vi "Basic Example.vi"(11 "System Definition Configuration":T34={"System Definition Path"=path "C:/Users/Public/Documents/National Instruments/NI VeriStand 2024/Projects/SimpleSystemDef Example/SimpleSystemDef.nivssdf", "Targets"=[{"Target Settings"={"Name"="Controller", "Target Type"="Windows", "IPAddress"="localhost", "PrimaryControlLoopProcessor"=-2, "DataProcessingLoopProcessor"=-2, "DataProcessingLoopDecimation"=1, "DAQDigitalLinesDecimation"=1, "MaximumStreamedChannels"=512, "ExecutionMode"=0, "FilterDAQErrors"=FALSE, "FilterWatchdogErrors"=FALSE, "FPGAScanInterfaceMode"=0, "TargetRate"=100.0}, "Chassises"=[{"Chassis Settings"={"Name"="Controller", "Master Chassis"={"Type"=enum."None", "DAQ Name"="", "clkSrc"=0, "activeEdge"=10280, "exportClk"=0, "exportClkToLine"=0, "triggerLine"=10171, "triggerSlope"=0, "startTrigger"=0, "startTriggerLine"=0}}, "DAQ Boards"=[{"Name"="DAQ1", "Description"="", "InputConfiguration"=10106, "TurnOffHWTimedSinglePointAI"=FALSE, "TurnOffHWTimedSinglePointAO"=FALSE, "DAQConversionRateOption"=0, "PortWidth"=8, "Analog Inputs"=[{"Name"="DAN0", "Units"="V", "InitialValue"=0.0, "HighLevel"=10.0, "LowLevel"=-10.0, "Channel"=0, "ChannelType"=0, "Alias Name"=""}, {"Name"="DAN1", "Units"="V", "InitialValue"=0.0, "HighLevel"=10.0, "LowLevel"=-10.0, "Channel"=1, "ChannelType"=0, "Alias Name"=""}], "Analog Outputs"=[{"Name"="DON0", "Units"="V", "InitialValue"=0.0, "HighLevel"=10.0, "LowLevel"=-10.0, "Channel"=0, "ChannelType"=0, "Alias Name"=""}, {"Name"="DON1", "Units"="V", "InitialValue"=0.0, "HighLevel"=10.0, "LowLevel"=-10.0, "Channel"=1, "ChannelType"=0, "Alias Name"=""}], "DIO Port Settings"=[{"portNumber"=0, "Inverted"=FALSE, "Digital Inputs"=[{"Name"="DIN0", "InitialValue"=FALSE, "DigitalLine"=0, "Alias Name"=""}, {"Name"="DIN1", "InitialValue"=FALSE, "DigitalLine"=2, "Alias Name"=""}], "Digital Outputs"=[{"Name"="DUN0", "InitialValue"=FALSE, "DigitalLine"=1, "Alias Name"=""}, {"Name"="DUN1", "InitialValue"=FALSE, "DigitalLine"=3, "Alias Name"=""}]}], "Counter Settings"={"Frequency Measurements"=[], "Period Measurements"=[], "Count Measurements"=[], "Position Measurements"=[]}}], "FPGA Boards"=[], "CAN Boards"=[]}], "Custom Devices"=[], "Models"=[], "User Channels"=[], "Calculated Channels"={"Formula Settings"=[], "Average Settings"=[], "Acceleration Settings"=[], "Maximum Settings"=[], "Minimum Settings"=[], "Peak and Valley Settings"=[], "Conditional Settings"=[]}, "Alarms"=[]}], "Aliases"=[], "System Mappings"={"Mapping Pairs"=[]}} {"Targets"."Alarms"."Priority" items=["Low", "Medium", "High"]; "Targets"."Alarms"."DefaultState" items=["Disabled", "Enabled"]; "Targets"."Alarms"."Mode" items=["Normal", "IndicateOnly"]; "Targets"."Target Settings"."FPGAScanInterfaceMode" items=["Use Current", "FPGA Mode", "Scan Mode"]; "Targets"."Target Settings"."ExecutionMode" items=["Parallel", "LowLatency"]; "Targets"."Chassises"."CAN Boards"."Log Files"."Operation" items=["ContinueLoggingInNewFile", "StopLogging"]; "Targets"."Chassises"."CAN Boards"."Log Files"."LimitType" items=["Footprint", "Time"]; "Targets"."Chassises"."CAN Boards"."Log Files"."TriggerType" items=["StartLoggingOnNonZero", "StartLoggingOnZero", "EnableLoggingWhenTriggerIsZero", "EnableLoggingWhenTriggerIsNonZero"]; "Targets"."Chassises"."CAN Boards"."Log Files"."Filter" items=["LogEntireBusTraffic", "ExcludeFrameIDs", "IncludeFrameIDs"]; "Targets"."Chassises"."CAN Boards"."Log Files"."DataLoggingFileType" items=["TDMS", "NCL"]; "Targets"."Chassises"."CAN Boards"."TransmitOrderType" items=["AsSubmitted", "ByIdentifier"]; "Targets"."Chassises"."CAN Boards"."TransceiverType" items=["HS", "LS", "SW"]; "Targets"."Chassises"."CAN Boards"."Termination" items=["Off", "On"]; "Targets"."Chassises"."CAN Boards"."Outgoing Frames"."Phase" items=["Unchanged", "Reset"]; "Targets"."Chassises"."CAN Boards"."Outgoing Frames"."TriggerType" items=["ChannelValueChange", "TriggerChannelNotZero", "ChannelValueChangeOrTriggerChannelNotZero"]; "Targets"."Chassises"."Chassis Settings"."Master Chassis"."startTriggerLine" items=["None", "PFI_0", "PFI_1", "PFI_2", "PFI_3", "PFI_4", "PFI_5", "PFI_6", "PFI_7", "PFI_8", "PFI_9", "PFI_10", "PFI_11", "PFI_12", "PFI_13", "PFI_14", "PFI_15", "RTSI_PXI_TRIG_0", "RTSI_PXI_TRIG_1", "RTSI_PXI_TRIG_2", "RTSI_PXI_TRIG_3", "RTSI_PXI_TRIG_4", "RTSI_PXI_TRIG_5", "RTSI_PXI_TRIG_6", "RTSI_PXI_TRIG_7"]; "Targets"."Chassises"."Chassis Settings"."Master Chassis"."startTrigger" items=["aiStartTrigger", "aoStartTrigger"]; "Targets"."Chassises"."Chassis Settings"."Master Chassis"."triggerSlope" items=["Falling"=10171, "Rising"=10280]; "Targets"."Chassises"."Chassis Settings"."Master Chassis"."triggerLine" items=["None", "PFI_0", "PFI_1", "PFI_2", "PFI_3", "PFI_4", "PFI_5", "PFI_6", "PFI_7", "PFI_8", "PFI_9", "PFI_10", "PFI_11", "PFI_12", "PFI_13", "PFI_14", "PFI_15", "RTSI_PXI_TRIG_0", "RTSI_PXI_TRIG_1", "RTSI_PXI_TRIG_2", "RTSI_PXI_TRIG_3", "RTSI_PXI_TRIG_4", "RTSI_PXI_TRIG_5", "RTSI_PXI_TRIG_6", "RTSI_PXI_TRIG_7"]; "Targets"."Chassises"."Chassis Settings"."Master Chassis"."exportClkToLine" items=["Default_RTSI_PXI_TRIG_0", "PFI_0", "PFI_1", "PFI_2", "PFI_3", "PFI_4", "PFI_5", "PFI_6", "PFI_7", "PFI_8", "PFI_9", "PFI_10", "PFI_11", "PFI_12", "PFI_13", "PFI_14", "PFI_15", "RTSI_PXI_TRIG_0", "RTSI_PXI_TRIG_1", "RTSI_PXI_TRIG_2", "RTSI_PXI_TRIG_3", "RTSI_PXI_TRIG_4", "RTSI_PXI_TRIG_5", "RTSI_PXI_TRIG_6", "RTSI_PXI_TRIG_7"]; "Targets"."Chassises"."Chassis Settings"."Master Chassis"."exportClk" items=["aiSampleClock", "aoSampleClock"]; "Targets"."Chassises"."Chassis Settings"."Master Chassis"."activeEdge" items=["Falling"=10171, "Rising"=10280]; "Targets"."Chassises"."Chassis Settings"."Master Chassis"."clkSrc" items=["Onboard10MHzClock", "PFI_0", "PFI_1", "PFI_2", "PFI_3", "PFI_4", "PFI_5", "PFI_6", "PFI_7", "PFI_8", "PFI_9", "PFI_10", "PFI_11", "PFI_12", "PFI_13", "PFI_14", "PFI_15", "RTSI_PXI_TRIG_0", "RTSI_PXI_TRIG_1", "RTSI_PXI_TRIG_2", "RTSI_PXI_TRIG_3", "RTSI_PXI_TRIG_4", "RTSI_PXI_TRIG_5", "RTSI_PXI_TRIG_6", "RTSI_PXI_TRIG_7"]; "Targets"."Chassises"."DAQ Boards"."Analog Outputs"."ChannelType" items=["Voltage", "Current"]; "Targets"."Chassises"."DAQ Boards"."Analog Inputs"."ChannelType" items=["Voltage", "Current"]; "Targets"."Chassises"."DAQ Boards"."DAQConversionRateOption" items=["Default", "Maximum"]; "Targets"."Chassises"."DAQ Boards"."InputConfiguration" items=["NRSE"=10078, "RSE"=10083, "Differential"=10106, "Pseudodifferential"=12529, "Default"=-1]}) -> (0 "error out":errorcluster)   [LabVIEW 2019, in "Simple SysDef API.lvlib"]
uses:
  <userlib>/SimpleSysDef/Simple SysDef API.lvlib
  <userlib>/SimpleSysDef/_SubVIs/Target Settings.ctl
  <userlib>/SimpleSysDef/_SubVIs/Add Target_Settings.ctl
  <userlib>/SimpleSysDef/_SubVIs/Add Target_Types.ctl
  <userlib>/SimpleSysDef/_SubVIs/Edit Chassis_Settings.ctl
  <userlib>/SimpleSysDef/_SubVIs/Add Chassis_DAQ Master Settings.ctl
  <userlib>/SimpleSysDef/_SubVIs/Add Chassis_Type.ctl
  <userlib>/SimpleSysDef/_SubVIs/Add DAQ Hardware_Settings.ctl
  <userlib>/SimpleSysDef/_SubVIs/Add DAQ Hardware_Analog Settings.ctl
  <userlib>/SimpleSysDef/_SubVIs/Add DAQ Hardware_Digital Port Settings.ctl
  <userlib>/SimpleSysDef/_SubVIs/Add DAQ Hardware_Digital Settings.ctl
  <userlib>/SimpleSysDef/_SubVIs/Add Frequency Measurement Channels_Settings.ctl
  <userlib>/SimpleSysDef/_SubVIs/Add Count Measurement Channels_Settings.ctl
  NationalInstruments.VeriStand.SystemDefinitionAPI
  <userlib>/SimpleSysDef/_SubVIs/Add Position Measurement Channels_Settings.ctl
  <userlib>/SimpleSysDef/_SubVIs/Add FPGA Hardware_Settings.ctl
  <userlib>/SimpleSysDef/_SubVIs/Add NI-XNET CAN Hardware_Port Settings.ctl
  <userlib>/SimpleSysDef/_SubVIs/Add NI-XNET CAN Hardware_Periodic Frame Settings.ctl
  <userlib>/SimpleSysDef/_SubVIs/Add NI-XNET CAN Hardware_Frame Settings.ctl
  <userlib>/SimpleSysDef/_SubVIs/Add NI-XNET CAN Hardware_Signal Settings.ctl
  <userlib>/SimpleSysDef/_SubVIs/Add NI-XNET CAN Hardware_Sporadic Frame Settings.ctl
  <userlib>/SimpleSysDef/_SubVIs/Add NI-XNET CAN Hardware_Add Log File_Settings.ctl
  <userlib>/SimpleSysDef/_SubVIs/Add Model_Settings.ctl
  <userlib>/SimpleSysDef/_SubVIs/Add User Channel_Settings.ctl
  <userlib>/SimpleSysDef/_SubVIs/Calculated Channels Cluster.ctl
  <userlib>/SimpleSysDef/_SubVIs/Add Calculate Channel_Formula_Settings.ctl
  <userlib>/SimpleSysDef/_SubVIs/Add Calculate Channel_Average_Settings.ctl
  <userlib>/SimpleSysDef/_SubVIs/Add Calculate Channel_Acceleration_Settings.ctl
  <userlib>/SimpleSysDef/_SubVIs/Add Calculate Channel_Maximum_Settings.ctl
  <userlib>/SimpleSysDef/_SubVIs/Add Calculate Channel_Peak and Valley_Settings.ctl
  <userlib>/SimpleSysDef/_SubVIs/Add Calculate Channel_Conditional_Settings.ctl
  <userlib>/SimpleSysDef/_SubVIs/Add Alarm_Settings.ctl
  <userlib>/SimpleSysDef/_SubVIs/Add Alias_Alias Settings.ctl
  <userlib>/SimpleSysDef/_SubVIs/Add System Mappings_Settings.ctl
  <userlib>/SimpleSysDef/_SubVIs/Add System Mappings_Settings_Channel Pairs.ctl
  <userlib>/SimpleSysDef/_SubVIs/Create New System Definition.vi
  <userlib>/SimpleSysDef/_SubVIs/Add Target.vi
  <userlib>/SimpleSysDef/_SubVIs/Add Model.vi
  <userlib>/SimpleSysDef/_SubVIs/Add System Mappings.vi
  <userlib>/SimpleSysDef/_SubVIs/Save and Close System Definition.vi
panel:
  in  "error in (no error)":errorcluster
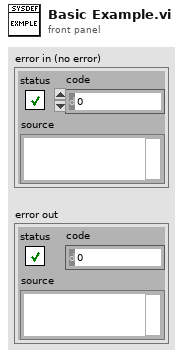
[diagram p1: front panel]
types:
  T1 = typedef "Simple SysDef API.lvlib/Target Settings.ctl" = cluster{"Target Settings":T2, "Chassises":cluster{"Chassis Settings":T4, "DAQ Boards":T7[], "FPGA Boards":T14[], "CAN Boards":T15[]}[], "Custom Devices":cluster{"Name":string, "Pre Initialization VI":path, "Pre Initialization VI Settings":cluster{"Control Name":string, "Value":variant}[], "Post Initialization VI":path, "Post Initialization VI Settings":cluster{"Control Name":string, "Value":variant}[]}[], "Models":T21[], "User Channels":T22[], "Calculated Channels":T23, "Alarms":T30[]}
  T2 = typedef "Simple SysDef API.lvlib/Add Target_Settings.ctl" = cluster{"Name":string, "Target Type":T3, "IPAddress":string, "PrimaryControlLoopProcessor":i32, "DataProcessingLoopProcessor":i32, "DataProcessingLoopDecimation":i32, "DAQDigitalLinesDecimation":u32, "MaximumStreamedChannels":i32, "ExecutionMode":i32, "FilterDAQErrors":bool, "FilterWatchdogErrors":bool, "FPGAScanInterfaceMode":u16, "TargetRate":dbl}
  T3 = typedef "Simple SysDef API.lvlib/Add Target_Types.ctl" = string
  T4 = typedef "Simple SysDef API.lvlib/Edit Chassis_Settings.ctl" = cluster{"Name":string, "Master Chassis":T5}
  T5 = typedef "Simple SysDef API.lvlib/Add Chassis_DAQ Master Settings.ctl" = cluster{"Type":T6, "DAQ Name":string, "clkSrc":i32, "activeEdge":i32, "exportClk":i32, "exportClkToLine":i32, "triggerLine":i32, "triggerSlope":i32, "startTrigger":i32, "startTriggerLine":i32}
  T6 = typedef "Simple SysDef API.lvlib/Add Chassis_Type.ctl" = enum16{"None", "DAQ", "FPGA", "Timing and Sync", "Automatic"}
  T7 = typedef "Simple SysDef API.lvlib/Add DAQ Hardware_Settings.ctl" = cluster{"Name":string, "Description":string, "InputConfiguration":i32, "TurnOffHWTimedSinglePointAI":bool, "TurnOffHWTimedSinglePointAO":bool, "DAQConversionRateOption":i32, "PortWidth":u16, "Analog Inputs":T8[], "Analog Outputs":T8[], "DIO Port Settings":T9[], "Counter Settings":cluster{"Frequency Measurements":T11[], "Period Measurements":T11[], "Count Measurements":T12[], "Position Measurements":T13[]}}
  T8 = typedef "Simple SysDef API.lvlib/Add DAQ Hardware_Analog Settings.ctl" = cluster{"Name":string, "Units":string, "InitialValue":dbl, "HighLevel":dbl, "LowLevel":dbl, "Channel":u32, "ChannelType":i32, "Alias Name":string}
  T9 = typedef "Simple SysDef API.lvlib/Add DAQ Hardware_Digital Port Settings.ctl" = cluster{"portNumber":u32, "Inverted":bool, "Digital Inputs":T10[], "Digital Outputs":T10[]}
  T10 = typedef "Simple SysDef API.lvlib/Add DAQ Hardware_Digital Settings.ctl" = cluster{"Name":string, "InitialValue":bool, "DigitalLine":u32, "Alias Name":string}
  T11 = typedef "Simple SysDef API.lvlib/Add Frequency Measurement Channels_Settings.ctl" = cluster{"Name":string, "Description":string, "Units":string, "Counter":u32, "DefaultValue":dbl, "Maximum":dbl, "Minimum":dbl, "Edge":i32, "Alias Name":string}
  T12 = typedef "Simple SysDef API.lvlib/Add Count Measurement Channels_Settings.ctl" = cluster{"Name":string, "Description":string, "Units":string, "Counter":u32, "DefaultValue":dbl, "CountDirection":i32, "Edge":i32, "ResetVariable":refnum<k24>, "Alias Name":string}
  T13 = typedef "Simple SysDef API.lvlib/Add Position Measurement Channels_Settings.ctl" = cluster{"Name":string, "Description":string, "Units":string, "Counter":u32, "DefaultValue":dbl, "Decoding":i32, "ZIndexMode":i32, "Alias Name":string}
  T14 = typedef "Simple SysDef API.lvlib/Add FPGA Hardware_Settings.ctl" = cluster{"Path":path, "RIO Name":string, "Aliases":cluster{"Relative Node Path":string, "Alias Name":string}[]}
  T15 = typedef "Simple SysDef API.lvlib/Add NI-XNET CAN Hardware_Port Settings.ctl" = cluster{"Name":string, "Database Name":string, "PortNumber":u16, "ClusterName":string, "BaudRate":u32, "InlineIncoming":bool, "IncomingRate":u32, "InlineOutgoing":bool, "OutgoingRate":u32, "Termination":i32, "Echo":bool, "InputStreamQueueSize":u32, "CANBusOff":bool, "CANBusOffRate":u32, "TransceiverType":i32, "TransmitOrderType":i32, "Cyclic Frames":T16[], "Outgoing Frames":T19[], "Incoming Frames":T17[], "Log Files":T20[]}
  T16 = typedef "Simple SysDef API.lvlib/Add NI-XNET CAN Hardware_Periodic Frame Settings.ctl" = cluster{"Frame Settings":T17, "Trigger Node Path":string, "TriggerType":i32, "Disable Node Path":string}
  T17 = typedef "Simple SysDef API.lvlib/Add NI-XNET CAN Hardware_Frame Settings.ctl" = cluster{"Name":string, "ID":u32, "PayloadLength":u32, "StartTimeOffset":dbl, "Enable64Bit":bool, "Signals":T18[]}
  T18 = typedef "Simple SysDef API.lvlib/Add NI-XNET CAN Hardware_Signal Settings.ctl" = cluster{"Name":string, "Description":string, "Units":string, "DefaultValue":dbl, "Alias Name":string}
  T19 = typedef "Simple SysDef API.lvlib/Add NI-XNET CAN Hardware_Sporadic Frame Settings.ctl" = cluster{"Frame Settings":T17, "Trigger Node Path":string, "TriggerType":i32, "Disable Node Path":string, "EnableSoftwareCyclicTrigger":bool, "TransmitTime":dbl, "Phase":i32}
  T20 = typedef "Simple SysDef API.lvlib/Add NI-XNET CAN Hardware_Add Log File_Settings.ctl" = cluster{"Name":string, "Filename":string, "Destination Folder":path, "NumberOfBytesToRead":u32, "DataLoggingFileType":i32, "TDMSGroupName":string, "TDMSChannelName":string, "Filter":i32, "FrameIDs":string[], "TriggerType":i32, "LimitType":i32, "LimitValue":u32, "Operation":i32, "Retriggerable":bool, "Trigger Node Path":string}
  T21 = typedef "Simple SysDef API.lvlib/Add Model_Settings.ctl" = cluster{"Name":string, "Description":string, "Path":path, "Processor":i32, "Decimation":i32, "InitialState":u16, "SegmentVectors":bool, "ImportParameters":bool, "ImportSignals":bool, "Group":i32}
  T22 = typedef "Simple SysDef API.lvlib/Add User Channel_Settings.ctl" = cluster{"Name":string, "Description":string, "Units":string, "DefaultValue":dbl, "Alias Name":string}
  T23 = typedef "Simple SysDef API.lvlib/Calculated Channels Cluster.ctl" = cluster{"Formula Settings":T24[], "Average Settings":T25[], "Acceleration Settings":T26[], "Maximum Settings":T27[], "Minimum Settings":T27[], "Peak and Valley Settings":T28[], "Conditional Settings":T29[]}
  T24 = typedef "Simple SysDef API.lvlib/Add Calculate Channel_Formula_Settings.ctl" = cluster{"Name":string, "Description":string, "Formula":string, "Variable Node Paths":string[], "Alias Name":string}
  T25 = typedef "Simple SysDef API.lvlib/Add Calculate Channel_Average_Settings.ctl" = cluster{"Name":string, "Description":string, "NumberOfPoints":u32, "Channel Node Path":string, "Alias Name":string}
  T26 = typedef "Simple SysDef API.lvlib/Add Calculate Channel_Acceleration_Settings.ctl" = cluster{"Name":string, "Description":string, "Units":string, "Channel to Analyze":string, "Channel for Velocity":string, "Alias Name":string}
  T27 = typedef "Simple SysDef API.lvlib/Add Calculate Channel_Maximum_Settings.ctl" = cluster{"Name":string, "Description":string, "X Constant":dbl, "X Channel Node":string, "Y Constant":dbl, "Y Channel Node":string, "Alias Name":string}
  T28 = typedef "Simple SysDef API.lvlib/Add Calculate Channel_Peak and Valley_Settings.ctl" = cluster{"Name":string, "Description":string, "Channel to Analyze Node Path":string, "Channel to Valley Node Path":string, "Channel to Offset Node Path":string, "Reset":u32, "Hysteresis":dbl, "Alias Name":string}
  T29 = typedef "Simple SysDef API.lvlib/Add Calculate Channel_Conditional_Settings.ctl" = cluster{"Name":string, "Description":string, "ComparisonMode":u16, "Channel to Check Node Path":string, "Y Constant":dbl, "Y Channel Node":string, "If True Constant":dbl, "If True Channel Node Path":string, "Else Constant ":dbl, "Else Channel Node Path":string, "Alias Name":string}
  T30 = typedef "Simple SysDef API.lvlib/Add Alarm_Settings.ctl" = cluster{"Name":string, "Description":string, "Alarm Channel Node Path":string, "UpperLimit":dbl, "Upper Limit Channel Node Path":string, "LowerLimit":dbl, "Lower Limit Channel Node Path":string, "Alarm Action Node Path":string, "Mode":i32, "DefaultState":i32, "Priority":i32, "Delay":dbl, "TripMessage":string, "GroupNumber":u32}
  T31 = typedef "Simple SysDef API.lvlib/Add Alias_Alias Settings.ctl" = cluster{"Name":string, "Description":string, "LinkedChannelPath":string}
  T32 = typedef "Simple SysDef API.lvlib/Add System Mappings_Settings.ctl" = cluster{"Mapping Pairs":T33[]}
  T33 = typedef "Simple SysDef API.lvlib/Add System Mappings_Settings_Channel Pairs.ctl" = cluster{"channelPathSources":string, "channelPathDestinations":string}
  T34 = cluster{"System Definition Path":path, "Targets":T1[], "Aliases":T31[], "System Mappings":T32}
  T35 = typedef "Simple SysDef API.lvlib/System Definition Reference.ctl" = refnum<k24>
  T36 = cluster{"Chassis Settings":T4, "DAQ Boards":T7[], "FPGA Boards":T14[], "CAN Boards":T15[]}[]
  T37 = cluster{"Name":string, "Pre Initialization VI":path, "Pre Initialization VI Settings":cluster{"Control Name":string, "Value":variant}[], "Post Initialization VI":path, "Post Initialization VI Settings":cluster{"Control Name":string, "Value":variant}[]}[]
  T38 = typedef "Simple SysDef API.lvlib/Target Node Paths.ctl" = cluster{"Hardware":string, "Custom Devices":string, "Simulation Models":string, "User Channels":string, "Calculated Channels":string, "Stimulus":string, "Alarms":string, "Procedures":string}
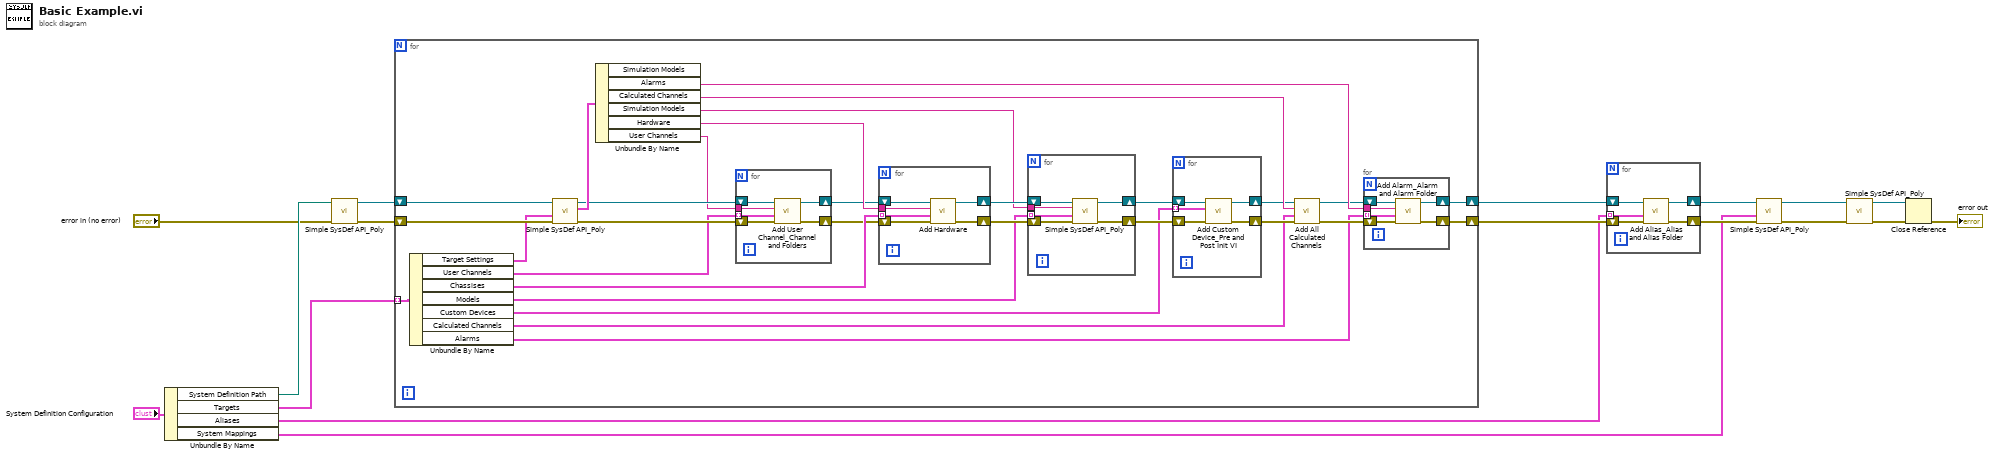
[diagram p0: block diagram]
diagram:
  n1 = Unbundle By Name("System Definition Configuration") -> ("System Definition Path"=w5:path, "Targets"=w4:T1[], "Aliases"=w3:T31[], "System Mappings"=w2:T32)
  n2 = call-poly <userlib>:"Simple SysDef API_Poly.vi"("error in (no error)"="error in (no error)", "path"=w5) -> ("error out"=w17:errorcluster, "SysDef Ref"=w16:T35)  [unwired: 7 in, 1 out]
  n3 = for {
    shift-right: [w39] -> w11
    shift-left: w16 -> [w41]
    shift-right: [w38] -> w12
    shift-left: w17 -> [w47]
    tunnel: w4 -> [w43] mode=indexing
    n4 = Unbundle By Name(w43) -> ("Target Settings"=w44:T2, "User Channels"=w22:T22[], "Chassises"=w42:T36, "Models"=w23:T21[], "Custom Devices"=w24:T37, "Calculated Channels"=w19:T23, "Alarms"=w18:T30[])
    n5 = call-poly <userlib>:"Simple SysDef API_Poly.vi"("error in (no error)"=w47, "Settings"=w44, "SysDef Ref"=w41) -> ("error out"=w33:errorcluster, "Target Node Paths"=w46:T38, "SysDef Ref Out"=w30:T35)  [unwired: 6 in]
    n6 = Unbundle By Name(w46) -> ("Alarms"=w37:string, "Calculated Channels"=w40:string, "Simulation Models"=w34:string, "Hardware"=w45:string, "User Channels"=w29:string)  [unwired: 1 out]
    n7 = for {
      tunnel: w29 -> [w60]
      shift-right: [w63] -> w32
      shift-left: w33 -> [w64]
      shift-right: [w62] -> w31
      shift-left: w30 -> [w61]
      tunnel: w22 -> [w59] mode=indexing
      n8 = call <userlib>:"Add User Channel_Channel and Folders.vi"("error in (no error)"=w64, "User Channel Settings"=w59, "Base Node Path"=w60, "SysDef Ref"=w61) -> ("error out"=w63:errorcluster, "SysDef Ref Out"=w62:T35)  [unwired: 6 in]
    }
    n9 = for {
      tunnel: w45 -> [w75]
      tunnel: w42 -> [w74] mode=indexing
      shift-right: [w72] -> w35
      shift-left: w31 -> [w73]
      shift-right: [w71] -> w36
      shift-left: w32 -> [w76]
      n10 = call <userlib>:"Add Hardware.vi"("error in (no error)"=w76, "Chassis Settings"=w74, "Hardware"=w75, "System Definition Ref"=w73) -> ("error out"=w71:errorcluster, "System Definition Ref"=w72:T35)  [unwired: 6 in]
    }
    n11 = for {
      tunnel: w34 -> [w69]
      shift-right: [w66] -> w28
      shift-left: w35 -> [w68]
      shift-right: [w67] -> w26
      shift-left: w36 -> [w70]
      tunnel: w23 -> [w65] mode=indexing
      n12 = call-poly <userlib>:"Simple SysDef API_Poly.vi"("error in (no error)"=w70, "Settings"=w65, "Base Node Path"=w69, "SysDef Ref"=w68) -> ("error out"=w67:errorcluster, "SysDef Ref Out"=w66:T35)  [unwired: 5 in, 1 out]
    }
    n13 = for {
      tunnel: w24 -> [w54] mode=indexing
      shift-right: [w57] -> w27
      shift-left: w28 -> [w58]
      shift-right: [w55] -> w25
      shift-left: w26 -> [w56]
      n14 = call <userlib>:"Add Custom Device_Pre and Post Init VI.vi"("error in (no error)"=w56, "Custom Device Settings"=w54, "System Definition Ref"=w58) -> ("error out"=w55:errorcluster, ".NET Refnum out"=w57:T35)  [unwired: 7 in]
    }
    n15 = call <userlib>:"Add All Calculated Channels.vi"("error in (no error)"=w25, "Calculated Channels Settings"=w19, "Calculated Channels"=w40, "System Definition Ref"=w27) -> ("error out"=w21:errorcluster, ".NET Refnum out"=w20:T35)  [unwired: 6 in]
    n16 = for {
      tunnel: w37 -> [w51]
      shift-right: [w53] -> w39
      shift-left: w20 -> [w49]
      shift-right: [w52] -> w38
      shift-left: w21 -> [w50]
      tunnel: w18 -> [w48] mode=indexing
      n17 = call <userlib>:"Add Alarm_Alarm and Alarm Folder.vi"("error in (no error)"=w50, "Alarm Settings"=w48, "Base Node Path"=w51, "SysDef Ref"=w49) -> ("error out"=w52:errorcluster, "SysDef Ref Out"=w53:T35)  [unwired: 6 in]
    }
  }
  n18 = for {
    shift-right: [w79] -> w10
    shift-left: w12 -> [w81]
    shift-right: [w78] -> w9
    shift-left: w11 -> [w80]
    tunnel: w3 -> [w77] mode=indexing
    n19 = call <userlib>:"Add Alias_Alias and Alias Folder.vi"("error in (no error)"=w81, "Alias Settings"=w77, "SysDef Ref"=w80) -> ("error out"=w79:errorcluster, "SysDef Ref Out"=w78:T35)  [unwired: 7 in]
  }
  n20 = call-poly <userlib>:"Simple SysDef API_Poly.vi"("error in (no error)"=w10, "Settings"=w2, "SysDef Ref"=w9) -> ("error out"=w8:errorcluster, "SysDef Ref Out"=w7:T35)  [unwired: 7 in]
  n21 = call-poly <userlib>:"Simple SysDef API_Poly.vi"("error in (no error)"=w8, "SysDef Ref"=w7) -> ("error out"=w15:errorcluster, "SysDef Ref out"=w13:T35)  [unwired: 8 in]
  n22 = Close Reference(reference=w13, error in (no error)=w15) -> (error out=→"error out":errorcluster)
